vi "Videos.vi"() -> ()   [LabVIEW 2019]
panel:
  in  "Video options":i32(listbox)
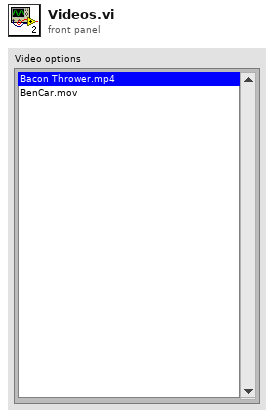
[diagram p1: front panel]
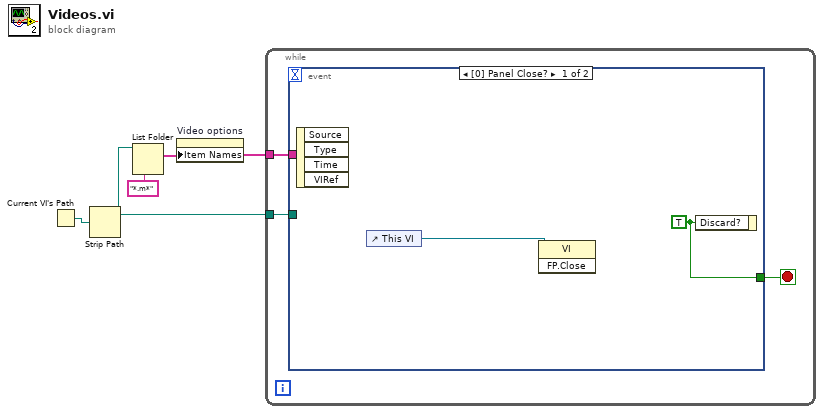
[diagram p0: block diagram]
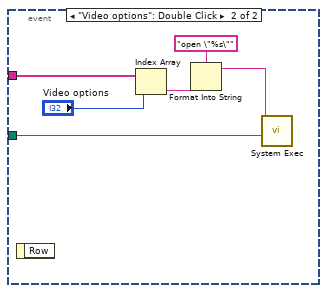
[diagram p2: hidden frame]
diagram:
  n1 = Current VI's Path() -> (path=w4:path)
  n2 = Strip Path(path=w4) -> (stripped path=w1:path)  [unwired: 1 out]
  n3 = List Folder(path=w1, pattern="*.m*") -> (filenames=w2:string[])  [unwired: 2 in, 3 out]
  n4 = property on="Video options" class="LstBox (strict)"("Item Names"=w2) -> ()  [unwired: 2 in, 2 out]
  n5 = while {
    tunnel: w2 -> [w6]
    tunnel: w1 -> [w5]
    stop <- w7 stop-if-true
    n6 = event shown="[0] Panel Close?" {
      selector: _ -> [_ _]
      dyn-events: _ -> [_ _]
      timeout: _ -> [_ _]
      tunnel: [w9 _] -> w7
      tunnel: w6 -> [_ w15]
      tunnel: w5 -> [_ w11]
      event Panel Close? {
        w9 = TRUE ("Discard?")
        n7 = event-data() -> ()  [unwired: 1 in, 4 out]
        n8 = control-ref of="This VI"() -> (w8:refnum<vi>)
        n9 = invoke class="VI" method="FP.Close"(reference=w8) -> ()  [unwired: 2 in, 3 out]
        n10 = event-data("Discard?"=w9) -> ()  [unwired: 1 in, 1 out]
      }
      event "Video options": Double Click {
        n11 = event-data() -> ()  [unwired: 1 in, 1 out]
        n12 = Index Array(array=w15, index="Video options") -> (element=w10:string)
        n13 = Format Into String(format string="open \"%s\"", w10) -> (resulting string=w12:string)  [unwired: 2 in, 1 out]
        n14 = call <vilib>:"System Exec.vi"("working directory"=w11, "command line"=w12) -> ()  [unwired: 6 in, 4 out]
      }
    }
  }
